vi "SmartSEM Remote API set SEM parameters.vi"(6 "Det Info":T1={"Brightness A"=40.0, "Contrast A"=26.0, "Detector B name"="ESB @ 1.0 kV", "Brightness B"=40.0, "Contrast B"=40.0, "Detector C name"="PMT @ 6.0", "Detector D name"="Detector D"}, 8 "error in":errorcluster, 9 "Scan Para":T2={"X resolution"=4096, "Y resolution"=2048, "X center (um)"=0.0, "Y center (um)"=0.0, "X size (V)"=20.0, "X size auto"=TRUE, "X stig"=0.0, "Y stig"=0.0, "X aln"=0.0, "Y aln"=0.0, "Scan rate (Hz)"=10000000, "Oversampling"=10, "Oversampling auto"=TRUE, "Frame line rampdown ratio"=0.1, "Pixel size (nm)"=5.0, "WD"=4.0} {"WD" format="%#_7g"; "Frame line rampdown ratio" min=-1 max=1 step=0.05 format="%.2g"; "Scan rate (Hz)" max=4000000 format="%.2e"}, 10 "SEM Options":T3={"GetInfo"=TRUE, "Set Det A para"=TRUE, "Set WD"=FALSE, "Set Mag"=TRUE, "Set stig"=FALSE, "Set aln"=FALSE, "Display"=TRUE, "Save"=TRUE, "8-bit"=TRUE, "Detector A"=TRUE, "Detector B"=FALSE, "Detector C"=FALSE, "Detector D"=FALSE, "Inverse A"=FALSE, "Inverse B"=FALSE, "Inverse C"=FALSE, "Inverse D"=FALSE, "Inverse PNG"=TRUE, "Freeze"=TRUE, "PNG only"=FALSE, "Upload"=FALSE, "Delete after upload"=FALSE}, 11 "Api in":refnum<k7>(container)) -> (0 "error out":errorcluster, 3 "Api out":refnum<k7>)   [LabVIEW 2018]
panel:
  out "Det A Type":string="InLens"
  out "Grid voltage":sgl
  out "Det B Type":string
  out "Set Mag":bool
  out "Set WD":bool
  out "Set aln":bool
  out "Set stig":bool
  out "Set Det para":bool
  out "Mag":sgl=285.0
  out "WD":sgl=0.0036
  out "Y aln":sgl=2.5
  out "X aln":sgl=1.5
  out "Y stig":sgl=1.0
  out "X stig":sgl=1.0
  out "Det A Contrast":sgl=45.0
  out "Det A Brightness":sgl=35.0
  out "Det B Contrast":sgl=40.0
  out "Det B Brightness":sgl=30.0
  # "Detector A"
  # "Det"
  # "after"
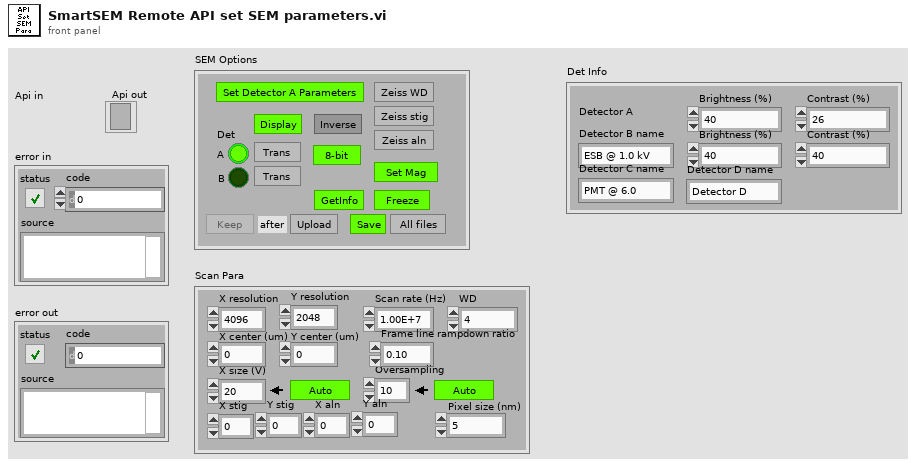
[diagram p1: front panel]
types:
  T1 = cluster{"Brightness A":dbl, "Contrast A":dbl, "Detector B name":string, "Brightness B":dbl, "Contrast B":dbl, "Detector C name":string, "Detector D name":string}
  T2 = cluster{"X resolution":u32, "Y resolution":u32, "X center (um)":sgl, "Y center (um)":sgl, "X size (V)":dbl, "X size auto":bool, "X stig":sgl, "Y stig":sgl, "X aln":sgl, "Y aln":sgl, "Scan rate (Hz)":u32, "Oversampling":u32, "Oversampling auto":bool, "Frame line rampdown ratio":sgl, "Pixel size (nm)":sgl, "WD":sgl}
  T3 = cluster{"GetInfo":bool, "Set Det A para":bool, "Set WD":bool, "Set Mag":bool, "Set stig":bool, "Set aln":bool, "Display":bool, "Save":bool, "8-bit":bool, "Detector A":bool, "Detector B":bool, "Detector C":bool, "Detector D":bool, "Inverse A":bool, "Inverse B":bool, "Inverse C":bool, "Inverse D":bool, "Inverse PNG":bool, "Freeze":bool, "PNG only":bool, "Upload":bool, "Delete after upload":bool}
  T4 = enum16{"SEM", "FIB", "Mill", "SEM + FIB", "Mill + SEM", "Drift SEM", "Drift FIB", "None", "Ext", "Ext + SEM"}
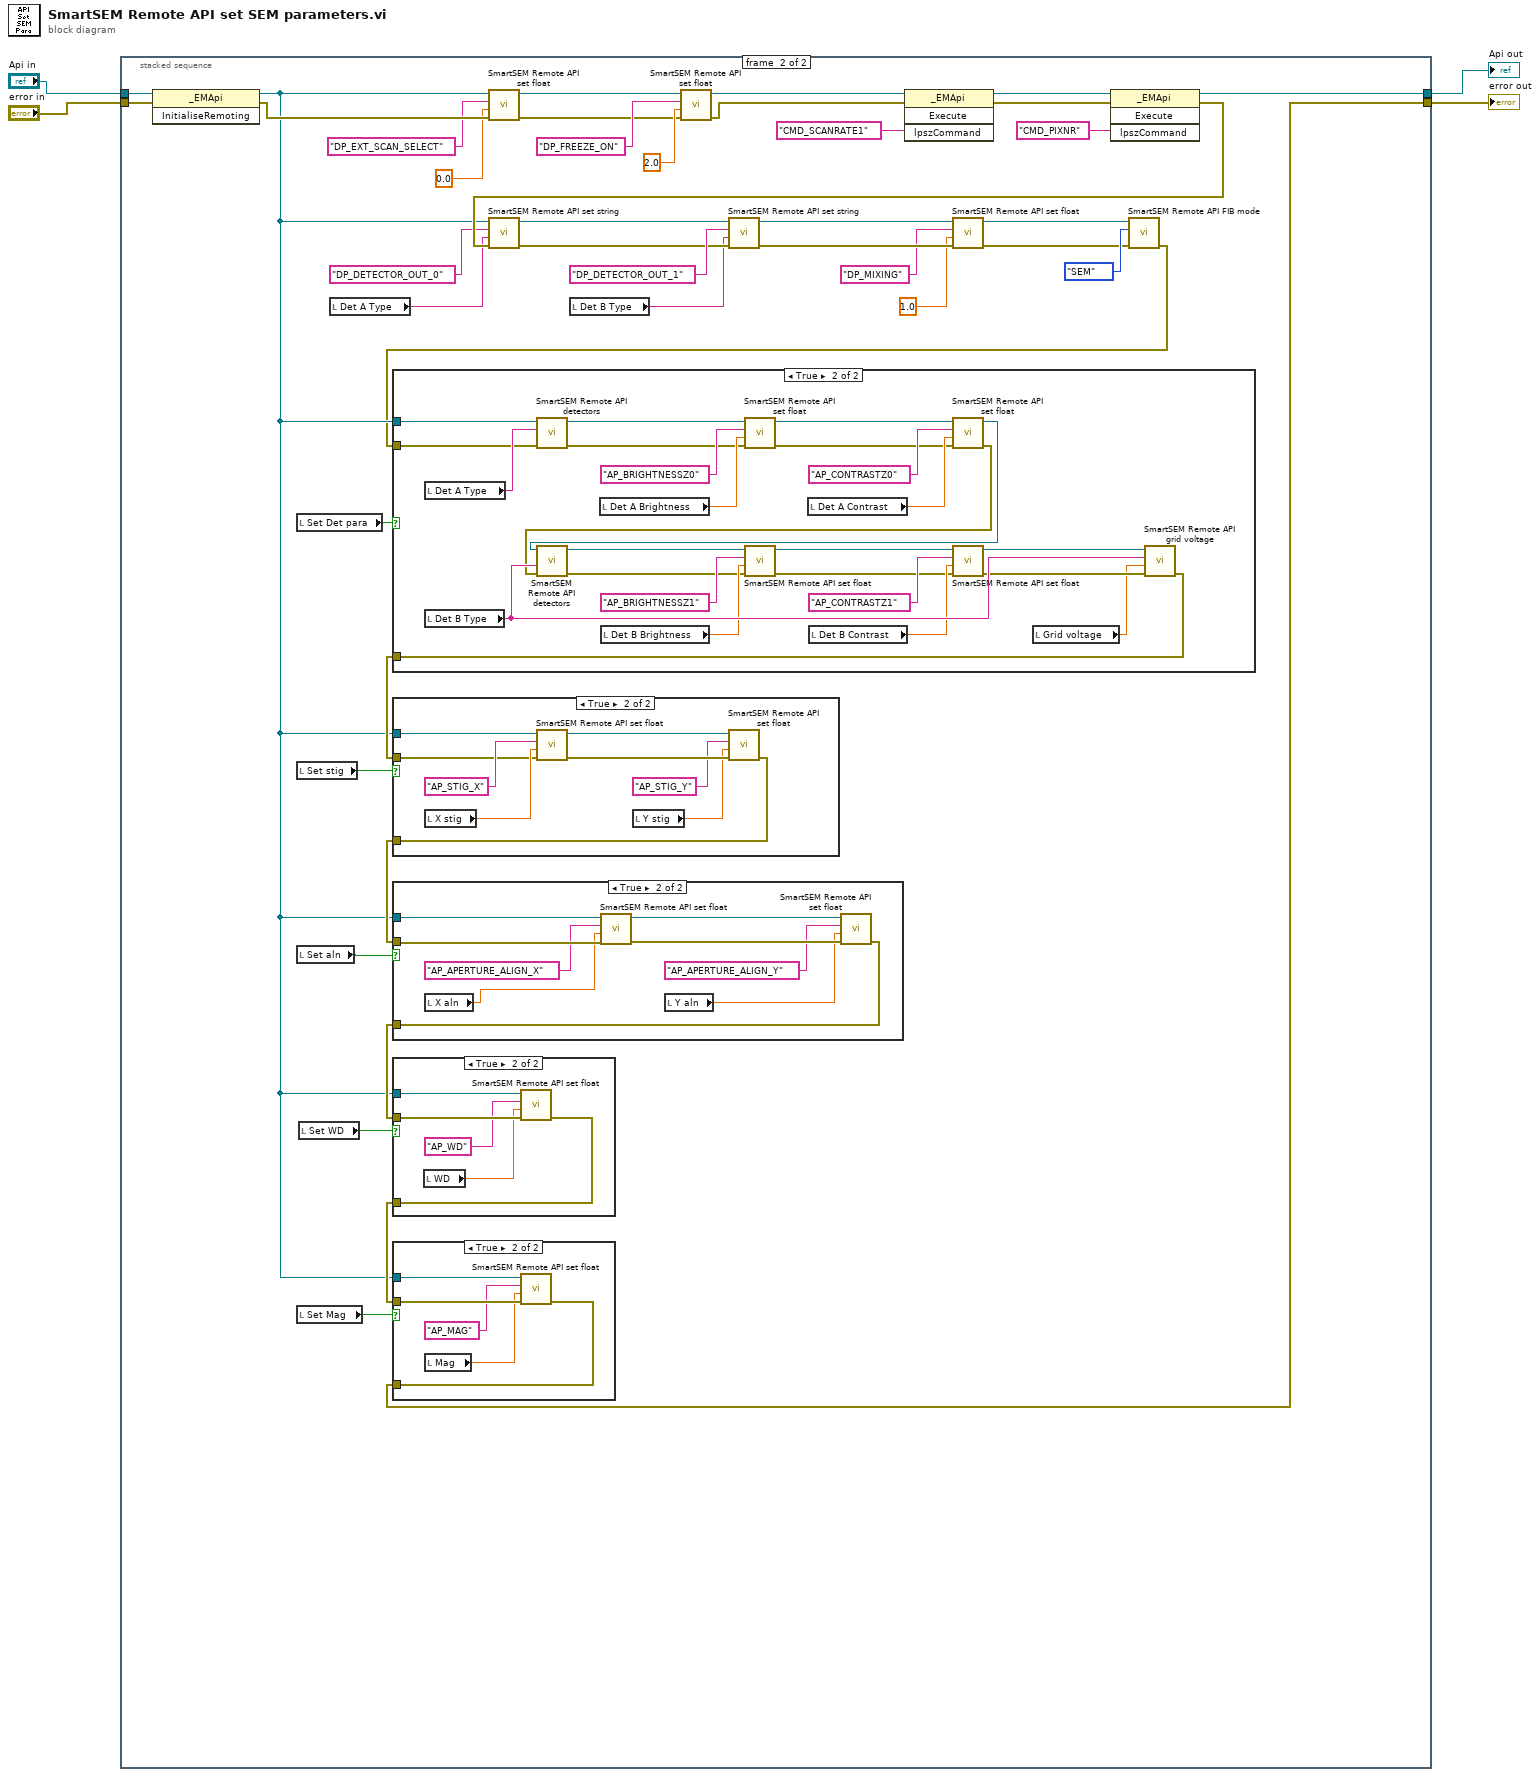
[diagram p0: block diagram]
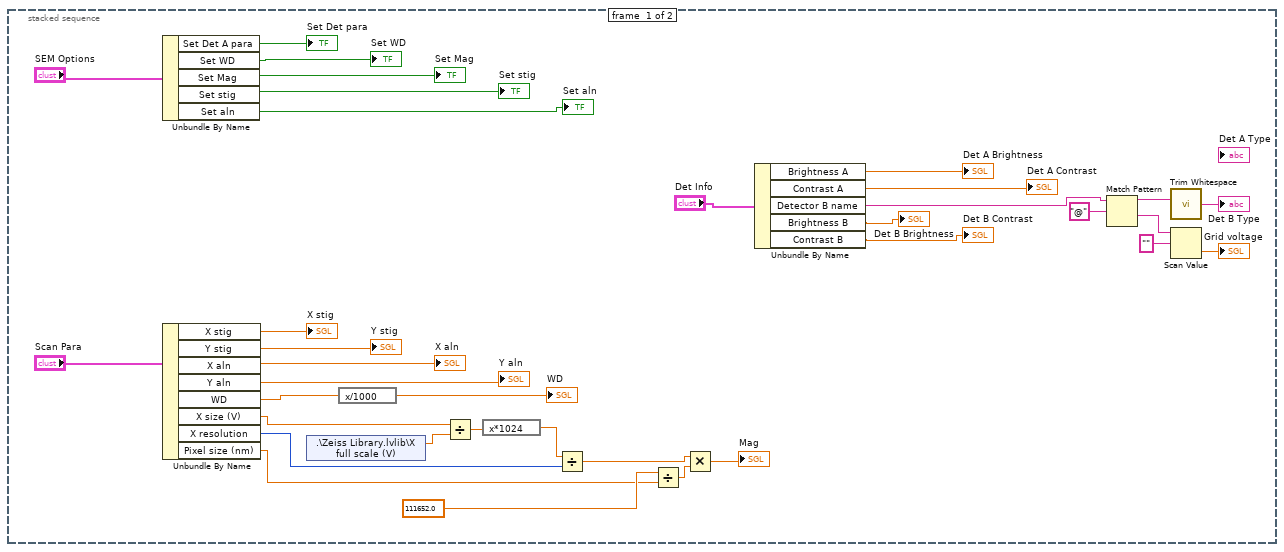
[diagram p2: hidden frame]
diagram:
  n1 = stacked-sequence {
    tunnel: [_ w74] -> w4
    tunnel: [_ w54] -> w1
    tunnel: "error in" -> [_ w73]
    tunnel: "Api in" -> [_ w72]
    frame #0 {
      n2 = Unbundle By Name("SEM Options") -> ("Set Det A para"=→"Set Det para":bool, "Set WD"=→"Set WD":bool, "Set Mag"=→"Set Mag":bool, "Set stig"=→"Set stig":bool, "Set aln"=→"Set aln":bool)
      n3 = Unbundle By Name("Scan Para") -> ("X stig"=→"X stig":sgl, "Y stig"=→"Y stig":sgl, "X aln"=→"X aln":sgl, "Y aln"=→"Y aln":sgl, "WD"=w28:sgl, "X size (V)"=w25:dbl, "X resolution"=w24:u32, "Pixel size (nm)"=w20:sgl)
      n4 = shared-variable ".\\Zeiss Library.lvlib\\X full scale (V)"() -> (w13:sgl)  [unwired: 1 in, 1 out]
      n5 = expression code="x/1000"(w28) -> (→"WD":sgl)
      n6 = Divide(x=w25, y=w13) -> (x/y=w26:dbl)
      n7 = expression code="x*1024"(w26) -> (w27:dbl)
      n8 = Divide(x=w27, y=w24) -> (x/y=w21:dbl)
      n9 = Divide(x=111652.0, y=w20) -> (x/y=w23:dbl)
      n10 = Multiply(x=w21, y=w23) -> (x*y=→"Mag":dbl)
      n11 = Unbundle By Name("Det Info") -> ("Brightness A"=→"Det A Brightness":dbl, "Contrast A"=→"Det A Contrast":dbl, "Detector B name"=w10:string, "Brightness B"=→"Det B Brightness":dbl, "Contrast B"=→"Det B Contrast":dbl)
      n12 = Match Pattern(string=w10, regular expression="@") -> (before substring=w9:string, after substring=w6:string)  [unwired: 1 in, 2 out]
      n13 = call <vilib>:"Trim Whitespace.vi"("string"=w9) -> ("trimmed string"=→"Det B Type":string)  [unwired: 1 in]
      n14 = Scan Value(string=w6, format string="") -> (value=→"Grid voltage":dbl)  [unwired: 1 in, 1 out]
    }
    frame #1 {
      n15 = invoke class="_EMApi" method="InitialiseRemoting"(reference=w72, error in=w73) -> (reference out=w58:refnum<k7>, error out=w60:errorcluster)  [unwired: 1 in, 1 out]
      n16 = local read "Set Det para"() -> (w80:bool)
      n17 = local read "Set stig"() -> (w79:bool)
      n18 = local read "Set aln"() -> (w78:bool)
      n19 = local read "Set Mag"() -> (w76:bool)
      n20 = local read "Set WD"() -> (w77:bool)
      n21 = local read "Det A Type"() -> (w65:string)
      n22 = call "SmartSEM Remote API set float.vi"("error in"=w60, "vValue"=sgl 0.0 ("Freeze on"), "lpszParam"="DP_EXT_SCAN_SELECT" ("lpszCommand"), "Api"=w58) -> ("error out"=w46:errorcluster, "Api out"=w47:refnum<k7>)  [unwired: 6 in]
      n23 = local read "Det B Type"() -> (w61:string)
      n24 = call "SmartSEM Remote API set float.vi"("error in"=w46, "vValue"=sgl 2.0 ("Freeze on"), "lpszParam"="DP_FREEZE_ON" ("lpszCommand"), "Api"=w47) -> ("error out"=w56:errorcluster, "Api out"=w57:refnum<k7>)  [unwired: 6 in]
      n25 = invoke class="_EMApi" method="Execute"(reference=w57, error in=w56, "lpszCommand"="CMD_SCANRATE1") -> (reference out=w51:refnum<k7>, error out=w50:errorcluster)  [unwired: 1 in, 2 out]
      n26 = invoke class="_EMApi" method="Execute"(reference=w51, error in=w50, "lpszCommand"="CMD_PIXNR") -> (reference out=w74:refnum<k7>, error out=w67:errorcluster)  [unwired: 1 in, 2 out]
      n27 = call "SmartSEM Remote API set string.vi"("error in"=w67, "vValue"=w65, "lpszParam"="DP_DETECTOR_OUT_0" ("lpszCommand"), "Api"=w58) -> ("error out"=w62:errorcluster, "Api out"=w63:refnum<k7>)  [unwired: 6 in]
      n28 = call "SmartSEM Remote API set string.vi"("error in"=w62, "vValue"=w61, "lpszParam"="DP_DETECTOR_OUT_1" ("lpszCommand"), "Api"=w63) -> ("error out"=w44:errorcluster, "Api out"=w45:refnum<k7>)  [unwired: 6 in]
      n29 = call "SmartSEM Remote API set float.vi"("error in"=w44, "vValue"=sgl 1.0 ("Freeze on"), "lpszParam"="DP_MIXING" ("lpszCommand"), "Api"=w45) -> ("error out"=w41:errorcluster, "Api out"=w40:refnum<k7>)  [unwired: 6 in]
      n30 = call "SmartSEM Remote API FIB mode.vi"("error in"=w41, "FIB mode"=T4."SEM", "Api"=w40) -> ("error out"=w48:errorcluster)  [unwired: 7 in, 1 out]
      n31 = case shown="True" w80 {
        tunnel: w58 -> [_ w131]
        tunnel: w48 -> [w114 w130]
        tunnel: [w114 w115] -> w71
        frame False {
        }
        frame True {
          n32 = local read "Det A Type"() -> (w140:string)
          n33 = local read "Det B Type"() -> (w129:string)
          n34 = call "SmartSEM Remote API detectors.vi"("error in"=w130, "Det A Type"=w140, "Api"=w131) -> ("error out"=w132:errorcluster, "Api out"=w133:refnum<k7>)  [unwired: 7 in]
          n35 = local read "Det A Brightness"() -> (w138:sgl)
          n36 = local read "Det B Brightness"() -> (w128:sgl)
          n37 = call "SmartSEM Remote API set float.vi"("error in"=w132, "vValue"=w138, "lpszParam"="AP_BRIGHTNESSZ0" ("lpszCommand"), "Api"=w133) -> ("error out"=w134:errorcluster, "Api out"=w139:refnum<k7>)  [unwired: 6 in]
          n38 = local read "Det A Contrast"() -> (w136:sgl)
          n39 = local read "Det B Contrast"() -> (w126:sgl)
          n40 = call "SmartSEM Remote API set float.vi"("error in"=w134, "vValue"=w136, "lpszParam"="AP_CONTRASTZ0" ("lpszCommand"), "Api"=w139) -> ("error out"=w116:errorcluster, "Api out"=w117:refnum<k7>)  [unwired: 6 in]
          n41 = call "SmartSEM Remote API detectors.vi"("error in"=w116, "Det B Type"=w129, "Api"=w117) -> ("error out"=w118:errorcluster, "Api out"=w119:refnum<k7>)  [unwired: 7 in]
          n42 = call "SmartSEM Remote API set float.vi"("error in"=w118, "vValue"=w128, "lpszParam"="AP_BRIGHTNESSZ1" ("lpszCommand"), "Api"=w119) -> ("error out"=w122:errorcluster, "Api out"=w124:refnum<k7>)  [unwired: 6 in]
          n43 = call "SmartSEM Remote API set float.vi"("error in"=w122, "vValue"=w126, "lpszParam"="AP_CONTRASTZ1" ("lpszCommand"), "Api"=w124) -> ("error out"=w121:errorcluster, "Api out"=w123:refnum<k7>)  [unwired: 6 in]
          n44 = local read "Grid voltage"() -> (w120:sgl)
          n45 = call "SmartSEM Remote API grid voltage.vi"("error in"=w121, "Grid voltage"=w120, "Det Type"=w129, "Api"=w123) -> ("error out"=w115:errorcluster)  [unwired: 6 in, 1 out]
        }
      }
      n46 = case shown="True" w79 {
        tunnel: w58 -> [_ w113]
        tunnel: w71 -> [w104 w105]
        tunnel: [w104 w108] -> w70
        frame False {
        }
        frame True {
          n47 = local read "X stig"() -> (w107:sgl)
          n48 = call "SmartSEM Remote API set float.vi"("error in"=w105, "vValue"=w107, "lpszParam"="AP_STIG_X" ("lpszCommand"), "Api"=w113) -> ("error out"=w111:errorcluster, "Api out"=w112:refnum<k7>)  [unwired: 6 in]
          n49 = local read "Y stig"() -> (w110:sgl)
          n50 = call "SmartSEM Remote API set float.vi"("error in"=w111, "vValue"=w110, "lpszParam"="AP_STIG_Y" ("lpszCommand"), "Api"=w112) -> ("error out"=w108:errorcluster)  [unwired: 6 in, 1 out]
        }
      }
      n51 = case shown="True" w78 {
        tunnel: w58 -> [_ w103]
        tunnel: w70 -> [w94 w102]
        tunnel: [w94 w95] -> w69
        frame False {
        }
        frame True {
          n52 = local read "X aln"() -> (w101:sgl)
          n53 = call "SmartSEM Remote API set float.vi"("error in"=w102, "vValue"=w101, "lpszParam"="AP_APERTURE_ALIGN_X" ("lpszCommand"), "Api"=w103) -> ("error out"=w98:errorcluster, "Api out"=w99:refnum<k7>)  [unwired: 6 in]
          n54 = local read "Y aln"() -> (w97:sgl)
          n55 = call "SmartSEM Remote API set float.vi"("error in"=w98, "vValue"=w97, "lpszParam"="AP_APERTURE_ALIGN_Y" ("lpszCommand"), "Api"=w99) -> ("error out"=w95:errorcluster)  [unwired: 6 in, 1 out]
        }
      }
      n56 = case shown="True" w77 {
        tunnel: w58 -> [_ w89]
        tunnel: w69 -> [w88 w93]
        tunnel: [w88 w92] -> w68
        frame False {
        }
        frame True {
          n57 = local read "WD"() -> (w90:sgl)
          n58 = call "SmartSEM Remote API set float.vi"("error in"=w93, "vValue"=w90, "lpszParam"="AP_WD" ("lpszCommand"), "Api"=w89) -> ("error out"=w92:errorcluster)  [unwired: 6 in, 1 out]
        }
      }
      n59 = case shown="True" w76 {
        tunnel: w58 -> [_ w87]
        tunnel: w68 -> [w82 w86]
        tunnel: [w82 w85] -> w54
        frame False {
        }
        frame True {
          n60 = local read "Mag"() -> (w84:sgl)
          n61 = call "SmartSEM Remote API set float.vi"("error in"=w86, "vValue"=w84, "lpszParam"="AP_MAG" ("lpszCommand"), "Api"=w87) -> ("error out"=w85:errorcluster)  [unwired: 6 in, 1 out]
        }
      }
    }
  }
  "Api out" <- w4
  "error out" <- w1
